vi "xz2mv.vi"(4 "error in (no error)":errorcluster, 5 "Cluster":T1) -> (0 "errorout":errorcluster, 1 "Array":waveform(i16)[](array[waveform]), 2 "time stamp":timestamp)   [LabVIEW 2010]
uses:
  lib/Global 2.vi
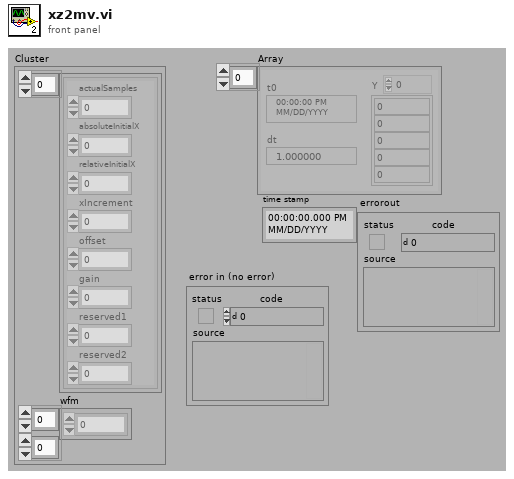
[diagram p1: front panel]
types:
  T1 = cluster{cluster{"actualSamples":i32, "absoluteInitialX":dbl, "relativeInitialX":dbl, "xIncrement":dbl, "offset":dbl, "gain":dbl, "reserved1":dbl, "reserved2":dbl}[], "wfm":i16[][]}
  T2 = cluster{"actualSamples":i32, "absoluteInitialX":dbl, "relativeInitialX":dbl, "xIncrement":dbl, "offset":dbl, "gain":dbl, "reserved1":dbl, "reserved2":dbl}[]
  T3 = cluster{"name":enum16{"sync", "phase_a", "phase_b", "phase_c", "ground"}, "num":i32, "Numeric":i32}[]
  T4 = enum16{"sync", "phase_a", "phase_b", "phase_c", "ground"}
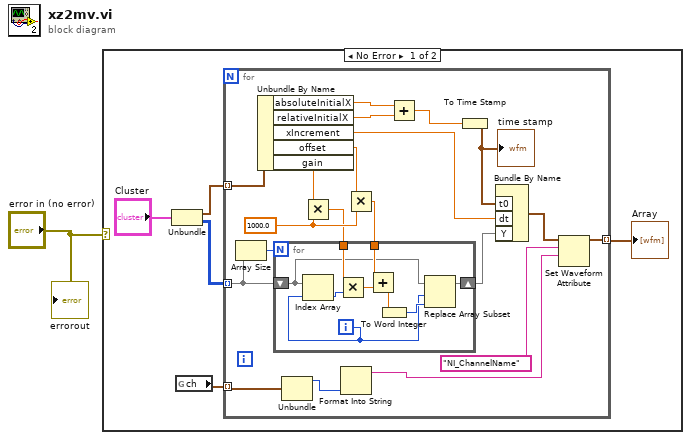
[diagram p0: block diagram]
diagram:
  n1 = case shown="No Error" "error in (no error)" {
    frame No Error {
      n2 = Unbundle("Cluster") -> (w5:T2, "wfm"=w6:i16[][])
      n3 = global read "Global 2.vi" "ch"() -> (w2:T3)
      n4 = for {
        tunnel: w5 -> [w24] mode=indexing
        tunnel: w6 -> [w11] mode=indexing
        tunnel: w2 -> [w14] mode=indexing
        tunnel: [w16] -> w3 mode=indexing
        w23 = 1000.0
        n5 = Array Size(array=w11) -> (size(s)=w10:i32)
        n6 = Unbundle By Name(w24) -> ("absoluteInitialX"=w9:dbl, "relativeInitialX"=w8:dbl, "xIncrement"=w19:dbl, "offset"=w25:dbl, "gain"=w26:dbl)
        n7 = Unbundle(w14) -> ("name"=w13:T4)  [unwired: 2 out]
        n8 = Multiply(x=w26, y=w23) -> (x*y=w21:dbl)
        n9 = Format Into String(w13) -> (resulting string=w12:string)  [unwired: 3 in, 1 out]
        n10 = Multiply(x=w25, y=w23) -> (x*y=w22:dbl)
        n11 = for {
          N: w10 -> [_]
          tunnel: w21 -> [w33]
          tunnel: w22 -> [w32]
          shift-right: [w28] -> w20
          shift-left: w11 -> [w30]
          i -> [w27]
          n12 = Index Array(array=w30, index=w27) -> (element=w31:i16)
          n13 = Multiply(x=w33, y=w31) -> (x*y=w35:dbl)
          n14 = Add(x=w32, y=w35) -> (x+y=w34:dbl)
          n15 = To Word Integer(number=w34) -> (16bit integer=w29:i16)
          n16 = Replace Array Subset(array=w30, new element=w29, index=w27) -> (w28:i16[])
        }
        n17 = Add(x=w9, y=w8) -> (x+y=w7:dbl)
        n18 = To Time Stamp(1:w7) -> (0:w18:timestamp)
        "time stamp" <- w18
        n19 = Bundle By Name("t0"=w18, "dt"=w19, "Y"=w20) -> (w17:waveform(i16))  [unwired: 1 in]
        n20 = Set Waveform Attribute(5:w12, 6:"NI_ChannelName" ("name"), 7:w17) -> (3:w16:waveform(i16))  [unwired: 1 in, 2 out]
      }
      "Array" <- w3
    }
    frame Error {
    }
  }
  "errorout" <- "error in (no error)"
